vi "Get Specific File Type Version Number.vi"(8 "Error In":errorcluster, 10 "Specific File Extension (e.g \"exe\", \"dll\" or \"lvlibp\")":string, 11 "Filepath":path) -> (0 "Error Out":errorcluster, 3 "File Version Number":string)   [LabVIEW 2023, in "Error Manager.lvlib"]
doc: "Retrieves the File Version of a specific file type (specific file extension)."
uses:
  Error Manager.lvlib
panel:
  # "Development\ncontrols/indicators useful for development and testing, but which are not outputs of the VI"
  # "Input\nInputs to the VI"
  # "Output\nOutputs of the VI"
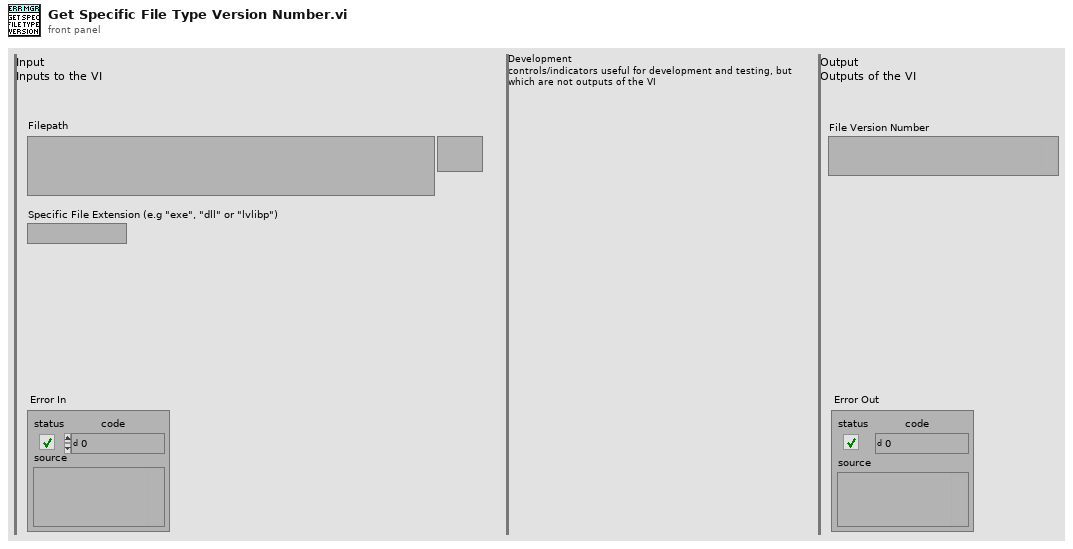
[diagram p1: front panel]
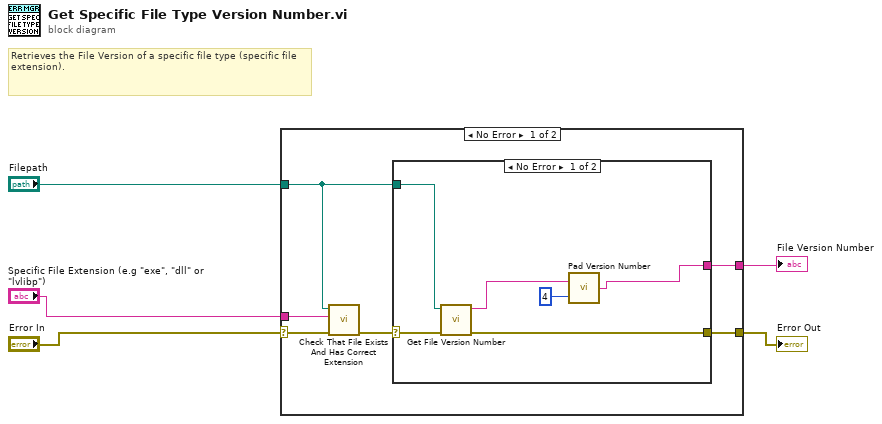
[diagram p0: block diagram]
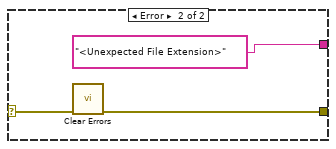
[diagram p2: hidden frame]
diagram:
  # "Retrieves the File Version of a specific file type (specific file extension)."
  n1 = case shown="No Error" "Error In" {
    selector: "Error In" -> [w11 w21]
    tunnel: [w9 w21] -> w4
    tunnel: "Filepath" -> [w7 _]
    tunnel: [w8 _] -> w2
    tunnel: "Specific File Extension (e.g \"exe\", \"dll\" or \"lvlibp\")" -> [w6 _]
    frame No Error {
      n2 = call "Check That File Exists And Has Correct Extension.vi"("error in"=w11, "Expected File Extension (case insensitive) (e.g \"txt\" or \"EXE\")"=w6, "Filepath"=w7) -> ("error out"=w10:errorcluster)  [unwired: 8 in]
      n3 = case shown="No Error" w10 {
        selector: w10 -> [w17 w20]
        tunnel: [w16 w19] -> w9
        tunnel: [w14 "<Unexpected File Extension>"] -> w8
        tunnel: w7 -> [w15 _]
        frame No Error {
          n4 = call "Get File Version Number.vi"("error in"=w17, "Filepath"=w15) -> ("error out"=w16:errorcluster, "File Version Number"=w13:string)  [unwired: 8 in]
          n5 = call "Pad Version Number.vi"("Desired minimum number of fields (Dflt = 4)"=4, "Input Version Number"=w13) -> ("Output Version Number (padded)"=w14:string)
        }
        frame Error {
          n6 = call <vilib>:"Clear Errors.vi"("error in (no error)"=w20) -> ("error out"=w19:errorcluster)  [unwired: 5 in, 1 out]
        }
      }
    }
    frame Error {
    }
  }
  "Error Out" <- w4
  "File Version Number" <- w2
